vi "solar_addon Voyager Packets.vi"(11 "Variant":variant) -> (0 "error out":errorcluster)   [LabVIEW 2018]
doc: "This SOLAR addon displays the packets registered with Voyager."
uses:
  solar/solar_ctl SOLAR Refnum.ctl
  voyager/solar_voy_def/solar_voy_def_ctl PATH.ctl
panel:
  in  "Export":bool
  in  "Automatic":bool
  in  "Update":bool
  in  "Tree":string(tree)
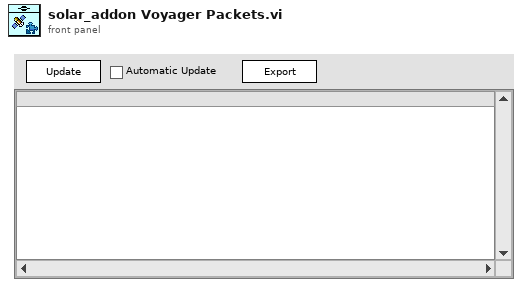
[diagram p1: front panel]
types:
  T1 = typedef "solar_ctl SOLAR Refnum.ctl" = refnum<k1>
  T2 = typedef "solar_voy_def_ctl PATH.ctl" = enum8{"..", "config", "config/data", "config/system", "config/targets", "config/targets/TARGET", "config/targets/TARGET/cmd_tlm", "config/targets/TARGET/lib", "config/targets/TARGET/screens", "config/tools", "config/tools/cmd_tlm_server", "config/tools/data_viewer", "config/tools/handbook_creator", "config/tools/launcher", "config/tools/limits_monitor", "config/tools/opengl_builder", "config/tools/script_runner", "config/tools/table_manager", "config/tools/test_runner", "config/tools/tlm_extractor", "config/tools/tlm_grapher", "config/tools/tlm_viewer", "lib", "outputs", "outputs/handbooks", "outputs/logs", "outputs/saved_config", "outputs/tables", "outputs/tmp", "procedures", "tools", "Launcher.bat", "config/system/system.txt", "config/targets/TARGET/cmd_tlm/TARGET_cmd.txt", "config/targets/TARGET/cmd_tlm/TARGET_tlm.txt", "config/targets/TARGET/cmd_tlm_server.txt", "config/targets/TARGET/target.txt", "config/tools/cmd_tlm_server/cmd_tlm_server.txt", "config/tools/data_viewer/data_viewer.txt", "config/tools/handbook_creator/handbook_creator.txt", "config/tools/launcher/launcher.txt", "config/tools/limits_monitor/limits_monitor.txt", "config/tools/opengl_builder/opengl_builder.txt", "config/tools/script_runner/script_runner.txt", "config/tools/table_manager/table_manager.txt", "config/tools/test_runner/test_runner.txt", "config/tools/tlm_extractor/tlm_extractor.txt", "config/tools/tlm_grapher/tlm_grapher.txt", "config/tools/tlm_viewer/tlm_viewer.txt"}
  T3 = typedef "solar_ctl SOLAR Global.ctl" = cluster{"Targets":T4[], "AppDir":path, "solar.ini":path, "ConfigsDir":path, "CosmosDir":path, "LogsDir":path, "ExePath":path, "ExeVersion":string, "PartNum":string, "AppSetup":string, "Title":string, "Main.ini":path, "Temp.ini":path, "vSOLAR":string, "Splash.png":string, "SplashWait":i32, "SOLARUE":refnum<user-event>, "VoyagerRefnum":T5, "QTimerRefnum":T6}
  T4 = typedef "solar_ctl Target Global.ctl" = cluster{"Target":string, "Q":refnum<queue>, "UE":refnum<user-event>, "VI":refnum<vi>, "Menu":refnum<k9>, "Data":refnum<data-value>, "Attributes":variant}
  T5 = typedef "solar_voy_ctl Voyager Refnum.ctl" = refnum<k1>
  T6 = typedef "solar_qtimer_ctl Refnum.ctl" = refnum<k1>
  T7 = typedef "solar_voy_ctl Voyager.ctl" = cluster{"PACKETS":T8[], "COSMOS_Root":path, "CMD_HDR":T13, "TLM_HDR":T13, "TCPs":T14[], "VoyagerIDOffset":cluster{"VoyagerIDOffset":u16[], "Target Names":string[]}}
  T8 = typedef "solar_voy_def_ctl PACKET.ctl" = cluster{"PACKET_ID":T9, "ENDIAN":enum8{"BIG", "LITTLE"}, "DESC":string, "HZRD":bool, "ITEMS":T10[], "NoExport":bool, "last_time":timestamp, "last_count":u32, "last_data":string}
  T9 = typedef "solar_voy_def_ctl PACKET_ID.ctl" = cluster{"ID":u16, "CMD":enum8{"CMD", "TLM"}, "TARGET":string, "PACKET":string}
  T10 = typedef "solar_voy_def_ctl ITEM.ctl" = cluster{"NAME":string, "OFFSET":i32, "SIZE":i32, "TYPE":T11, "EACH_SIZE":i32, "LVTYPE":T12, "MIN":dbl, "MAX":dbl, "DEFAULT":string, "DESC":string, "ID":bool, "MODIFIERS":variant, "last_value":variant}
  T11 = typedef "solar_voy_def_ctl ITEM TYPE.ctl" = enum8{"BLOCK", "INT", "UINT", "FLOAT", "STRING"}
  T12 = typedef "solar_type Item Type.ctl" = enum16{"NULL", "UNKNOWN", "CLUSTER", "I8", "I16", "I32", "I64", "U8", "U16", "U32", "U64", "U8_ENUM", "U16_ENUM", "U32_ENUM", "SGL", "DBL", "BOOLEAN", "STRING", "PATH", "VISA", "TAG", "TIME", "I8_1D", "I16_1D", "I32_1D", "I64_1D", "U8_1D", "U16_1D", "U32_1D", "U64_1D", "U8_ENUM_1D", "U16_ENUM_1D", "U32_ENUM_1D", "SGL_1D", "DBL_1D", "BOOLEAN_1D", "STRING_1D", "PATH_1D", "VISA_1D", "TAG_1D", "TIME_1D", "I8_2D", "I16_2D", "I32_2D", "I64_2D", "U8_2D", "U16_2D", "U32_2D", "U64_2D", "U8_ENUM_2D", "U16_ENUM_2D", "U32_ENUM_2D", "SGL_2D", "DBL_2D", "BOOLEAN_2D", "STRING_2D", "PATH_2D", "VISA_2D", "TAG_2D", "TIME_2D"}
  T13 = typedef "solar_voy_def_ctl HDR.ctl" = cluster{"ITEMS":T10[], "LENGTH_NAME":string, "LENGTH_VALUE_OFFSET":i32, "ID_NAME":string, "ENDIAN":enum8{"BIG", "LITTLE"}, "GUID_NAME":string, "DEFAULT_TARGET":string, "DEFAULT_PACKET":string, "DEFAULT_ERROR":string}
  T14 = typedef "solar_voy_ctl TCP.ctl" = cluster{"Connected":bool, "Port":u16, "Listener":refnum<k5>, "ServerIP":string, "TCP":refnum<k5>, "Setup":T15, "VIRefnum":refnum<vi>, "TARGETS_CMD":string[], "TARGETS_TLM":string[]}
  T15 = typedef "solar_voy_ctl Port Setup.ctl" = enum8{"SERVER", "CLIENT", "SERVER_CMD", "SERVER_TLM"}
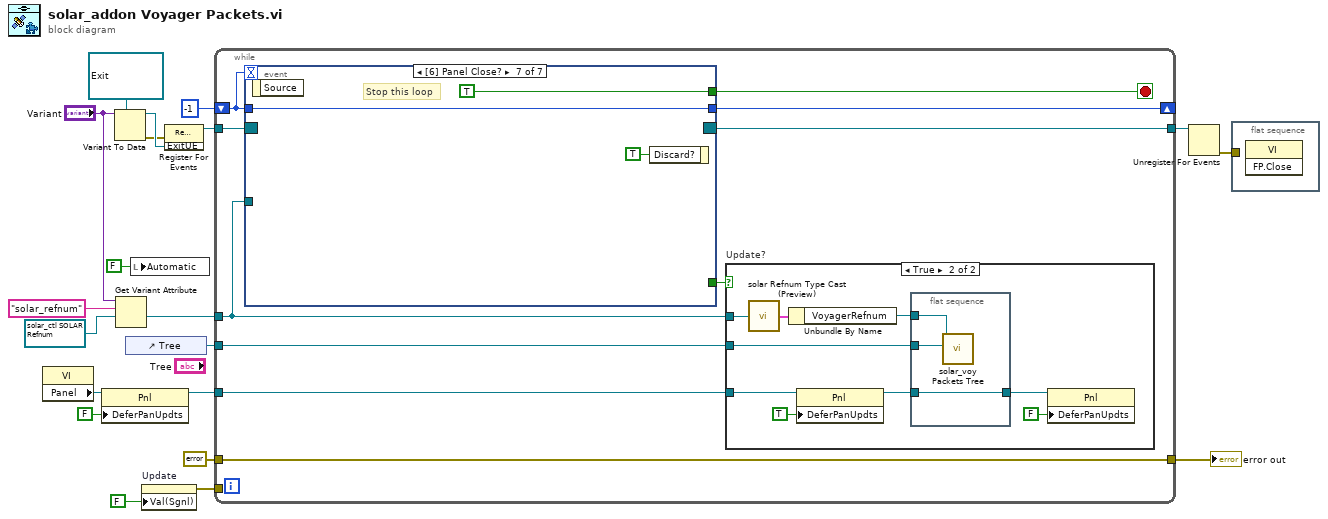
[diagram p0: block diagram]
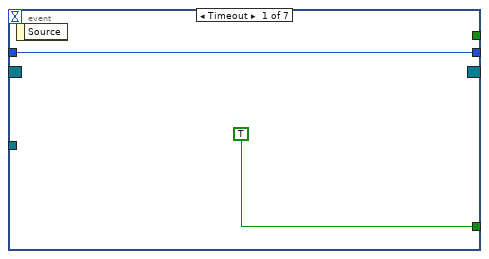
[diagram p2: hidden frame]
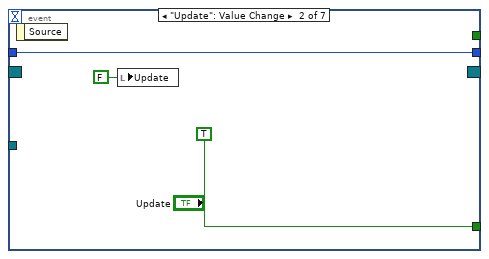
[diagram p3: hidden frame]
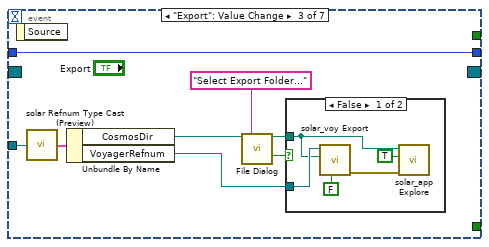
[diagram p4: hidden frame]
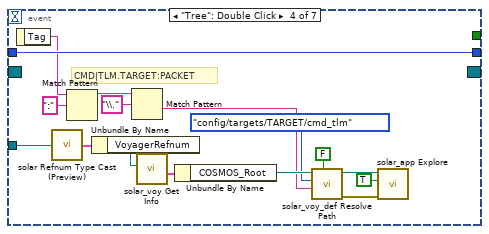
[diagram p6: hidden frame]
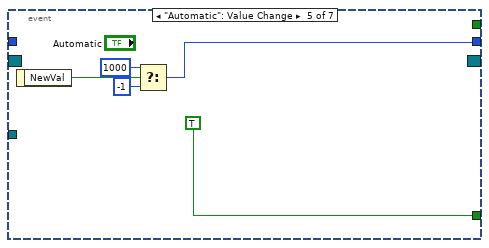
[diagram p7: hidden frame]
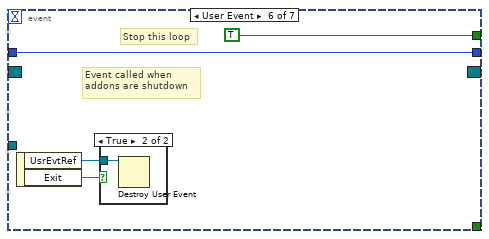
[diagram p8: hidden frame]
diagram:
  w15 = T1 refnum items=["solar"] ("SOLAR Refnum")
  n1 = property class="VI"() -> ("Panel"=w9:refnum<vi>)  [unwired: 2 in, 2 out]
  n2 = property class="Pnl"(reference=w9, "DeferPanUpdts"=FALSE ("Defer Panel Updates")) -> (reference out=w8:refnum<vi>)  [unwired: 1 in, 1 out]
  n3 = Variant To Data(type=refnum<user-event> refnum ("ExitUE"), Variant="Variant") -> (data=w17:refnum<user-event>, error out=w16:errorcluster)  [unwired: 1 in]
  n4 = Get Variant Attribute(Variant="Variant", name="solar_refnum", default value (empty Variant)=w15) -> (value=w12:T1)  [unwired: 1 in, 3 out]
  n5 = control-ref of="Tree"() -> (w11:refnum<vi>)
  n6 = local write "Automatic"(FALSE ("Automatic")) -> ()
  n7 = property on="Update" class="Bool (strict)"("Val(Sgnl)"=FALSE ("Update")) -> (error out=w5:errorcluster)  [unwired: 2 in, 1 out]
  n8 = register-events(error in=w16, w17) -> (reference out=w19:refnum<event-registration>)  [unwired: 1 in, 1 out]
  n9 = while {
    tunnel: w19 -> [w30]
    shift-right: [w26] -> _
    shift-left: -1 -> [w25]
    tunnel: w12 -> [w23]
    tunnel: w11 -> [w28]
    tunnel: w8 -> [w24]
    tunnel: w5 -> [_]
    tunnel: [w22] -> w4
    tunnel: [w21] -> w2
    tunnel: errorcluster {"status"=FALSE, "code"=0, "source"=""} ("error in (no error)") -> [w21]
    stop <- w29 stop-if-true
    n10 = event shown="[6] Panel Close?" {
      selector: w30 -> [_ _ _ _ _ _ _]
      dyn-events: [_ _ _ _ _ _ _] -> w22
      timeout: w25 -> [_ _ _ _ _ _ _]
      tunnel: [_ _ _ _ _ TRUE TRUE] -> w29
      tunnel: [TRUE TRUE _ _ TRUE _ _] -> w27
      tunnel: [w32 w34 w43 w64 w67 w72 w76] -> w26
      tunnel: w25 -> [w32 w34 w43 w64 _ w72 w76]
      tunnel: w23 -> [_ _ w41 w60 _ _ _]
      event Timeout {
        n11 = event-data() -> ()  [unwired: 1 in, 1 out]
      }
      event "Update": Value Change {
        n12 = event-data() -> ()  [unwired: 1 in, 1 out]
        n13 = local write "Update"(FALSE ("Update")) -> ()
      }
      event "Export": Value Change {
        n14 = event-data() -> ()  [unwired: 1 in, 1 out]
        n15 = call "solar Refnum Type Cast (Preview).vi"("Refnum"=w41) -> ("SOLAR"=w42:T3)  [unwired: 8 in]
        n16 = Unbundle By Name(w42) -> ("CosmosDir"=w37:path, "VoyagerRefnum"=w36:T5)
        n17 = call "File Dialog"("start path"=w37, "prompt"="Select Export Folder...") -> ("selected path"=w39:path, "cancelled"=w38:bool)  [unwired: 10 in, 2 out]
        n18 = case shown="False" w38 {
          tunnel: w39 -> [w45 _]
          tunnel: w36 -> [w47 _]
          frame False {
            n19 = call "solar_voy Export.vi"("Suppress Errors? (T)"=FALSE, "COSMOS Root (\"\" = Use Default)"=w45, "Voyager Refnum in"=w47) -> ("error out"=w46:errorcluster)  [unwired: 7 in, 1 out]
            n20 = call "solar_app Explore.vi"("error in (no error)"=w46, "Open Folder? (F)"=TRUE, "File or Folder Path"=w45) -> ()  [unwired: 8 in, 1 out]
          }
          frame True {
          }
        }
      }
      event "Tree": Double Click {
        # "CMD|TLM.TARGET:PACKET"
        n21 = event-data() -> ("Tag"=w63:string)  [unwired: 1 in]
        n22 = call "solar Refnum Type Cast (Preview).vi"("Refnum"=w60) -> ("SOLAR"=w61:T3)  [unwired: 8 in]
        n23 = Match Pattern(string=w63, regular expression=":") -> (before substring=w50:string)  [unwired: 1 in, 3 out]
        n24 = Unbundle By Name(w61) -> ("VoyagerRefnum"=w59:T5)
        n25 = Match Pattern(string=w50, regular expression="\\.") -> (after substring=w49:string)  [unwired: 1 in, 3 out]
        n26 = call "solar_voy Get Info.vi"("Voyager Refnum"=w59) -> ("Voyager"=w58:T7)  [unwired: 8 in, 2 out]
        n27 = Unbundle By Name(w58) -> ("COSMOS_Root"=w57:path)
        n28 = call "solar_voy_def Resolve Path.vi"("Create Folder? (T)"=FALSE, "TARGET"=w49, "PATH (..=Root)"=solar_voy_def_ctl_PATH."config/targets/TARGET/cmd_tlm", "COSMOS_ROOT"=w57) -> ("error out"=w52:errorcluster, "Resolved Path"=w53:path)  [unwired: 6 in]
        n29 = call "solar_app Explore.vi"("error in (no error)"=w52, "Open Folder? (F)"=TRUE, "File or Folder Path"=w53) -> ()  [unwired: 8 in, 1 out]
      }
      event "Automatic": Value Change {
        n30 = event-data() -> ("NewVal"=w69:bool)  [unwired: 1 in]
        n31 = Select(t=1000, s=w69, f=-1) -> (s? t:f=w67:i32)
      }
      event User Event {
        # "Stop this loop"
        # "Event called when\naddons are shutdown"
        n32 = event-data() -> ("UsrEvtRef"=w71:refnum<user-event>, "Exit"=w70:bool)  [unwired: 1 in]
        n33 = case shown="True" w70 {
          tunnel: w71 -> [_ w74]
          frame False {
          }
          frame True {
            n34 = Destroy User Event(user event=w74) -> ()  [unwired: 1 in, 1 out]
          }
        }
      }
      event Panel Close? {
        # "Stop this loop"
        n35 = event-data() -> ()  [unwired: 1 in, 1 out]
        n36 = event-data("Discard?"=TRUE) -> ()  [unwired: 1 in, 1 out]
      }
    }
    n37 = case "Update?" shown="True" w27 {
      tunnel: w23 -> [_ w84]
      tunnel: w28 -> [_ w83]
      tunnel: w24 -> [_ w81]
      frame False {
      }
      frame True {
        n38 = call "solar Refnum Type Cast (Preview).vi"("Refnum"=w84) -> ("SOLAR"=w86:T3)  [unwired: 8 in]
        n39 = Unbundle By Name(w86) -> ("VoyagerRefnum"=w85:T5)
        n40 = property class="Pnl"(reference=w81, "DeferPanUpdts"=TRUE ("Defer Panel Updates")) -> (reference out=w80:refnum<vi>)  [unwired: 1 in, 1 out]
        n41 = flat-sequence {
          tunnel: w85 -> [w89]
          tunnel: w83 -> [w88]
          tunnel: [w87] -> w78
          tunnel: w80 -> [w87]
          frame #0 {
            n42 = call "solar_voy Packets Tree.vi"("Tree Refnum"=w88, "Voyager Refnum in"=w89) -> ()  [unwired: 8 in, 2 out]
          }
        }
        n43 = property class="Pnl"(reference=w78, "DeferPanUpdts"=FALSE ("Defer Panel Updates")) -> ()  [unwired: 1 in, 2 out]
      }
    }
  }
  "error out" <- w2
  n44 = Unregister For Events(event registration refnum=w4) -> (error out=w3:errorcluster)  [unwired: 1 in]
  n45 = flat-sequence {
    tunnel: w3 -> [_]
    frame #0 {
      n46 = invoke class="VI" method="FP.Close"() -> ()  [unwired: 3 in, 3 out]
    }
  }
